vi "Wind tunnel coriolis accel calc.vi"(0 "Wind tunnel streamwise heading (deg)":dbl=90.7145, 5 "Wind tunnel streamwise elevation angle (deg)":dbl, 7 "Wind tunnel latitude (deg North of equator)":dbl=51.243148, 9 "Streamwise velocity component (m/s)":dbl=2.5, 11 "Earth angular velocity (rad/s)":dbl=7.292115e-05 format="%#.4g", 12 "Earth equatorial radius (km)":dbl=6378.137 format="%#.4g", 13 "Earth polar radius (km)":dbl=6356.7523 format="%#.4g", 14 "Wind tunnel streamwise fetch L (m)":dbl=20.0) -> (3 "Streamwise direction vector":dbl[](array[numeric])=[0.009724268343721, 0.999922245850074, -0.007806462663934707] format="%#_4g", 4 "Coriolis acceleration vector (m/s^2)":dbl[](array[numeric])=[0.00036457740038985066, -3.5455241526636534e-06, 0.0] format="%#.3e", 6 "Angle of coriolis acceleration from true North (deg)":dbl=141.23977334051196 format="%.2f", 8 "Angle of coriolis acceleration from true East (deg)":dbl=90.55718529475455 format="%.2f", 10 "Induced velocity from coriolis acceleration at L (mm/s)":dbl=2.916757121095013 format="%_3g", 15 "Induced displacement from coriolis acceleration at L (mm)":dbl=11.667028484380053 format="%_3g")   [LabVIEW 2013]
uses:
  <vilib>/Analysis/_algsub.llb/Real Vector Norm.vi
  <vilib>/Analysis/baseanly.llb/Unit Vector (DBL).vi
  <vilib>/Analysis/baseanly.llb/Real Dot Product.vi
  <vilib>/Analysis/NI_AALBase.lvlib
  <vilib>/Analysis/NI_AALPro.lvlib
panel:
  out "WGS84 Earth surface gravitational acceleration (m/s^2)":dbl=9.811808032478377
  out "Earth surface tangential velocity (m/s)":dbl=290.56938190964064
  out "WGS84 Geoid radius (km)":dbl=6365.175727728627
  # "Paul Nathan 19/02/2014"
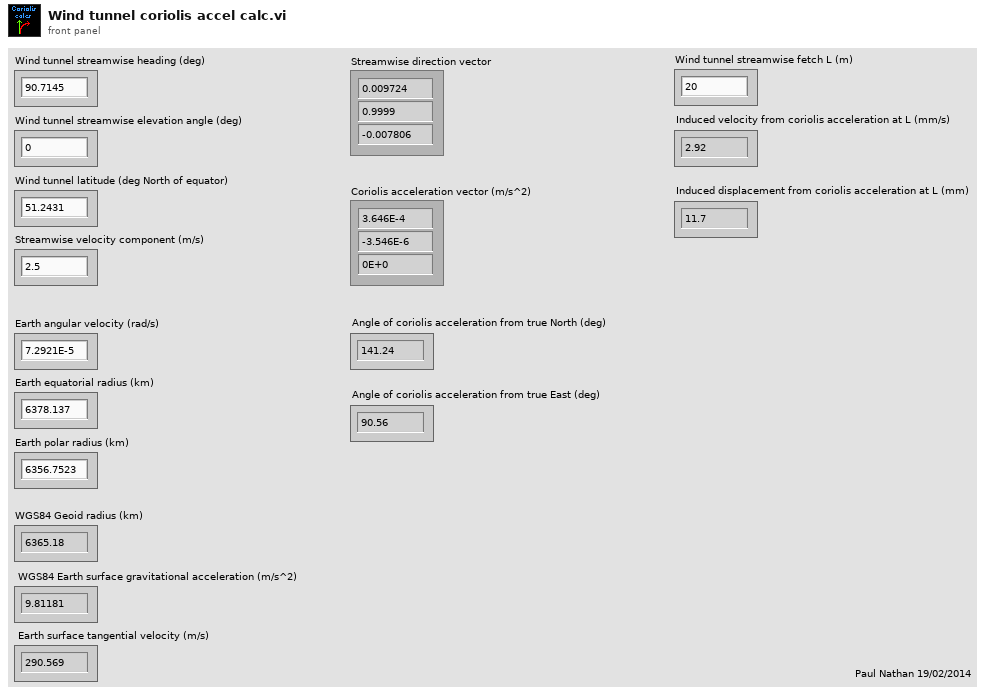
[diagram p1: front panel]
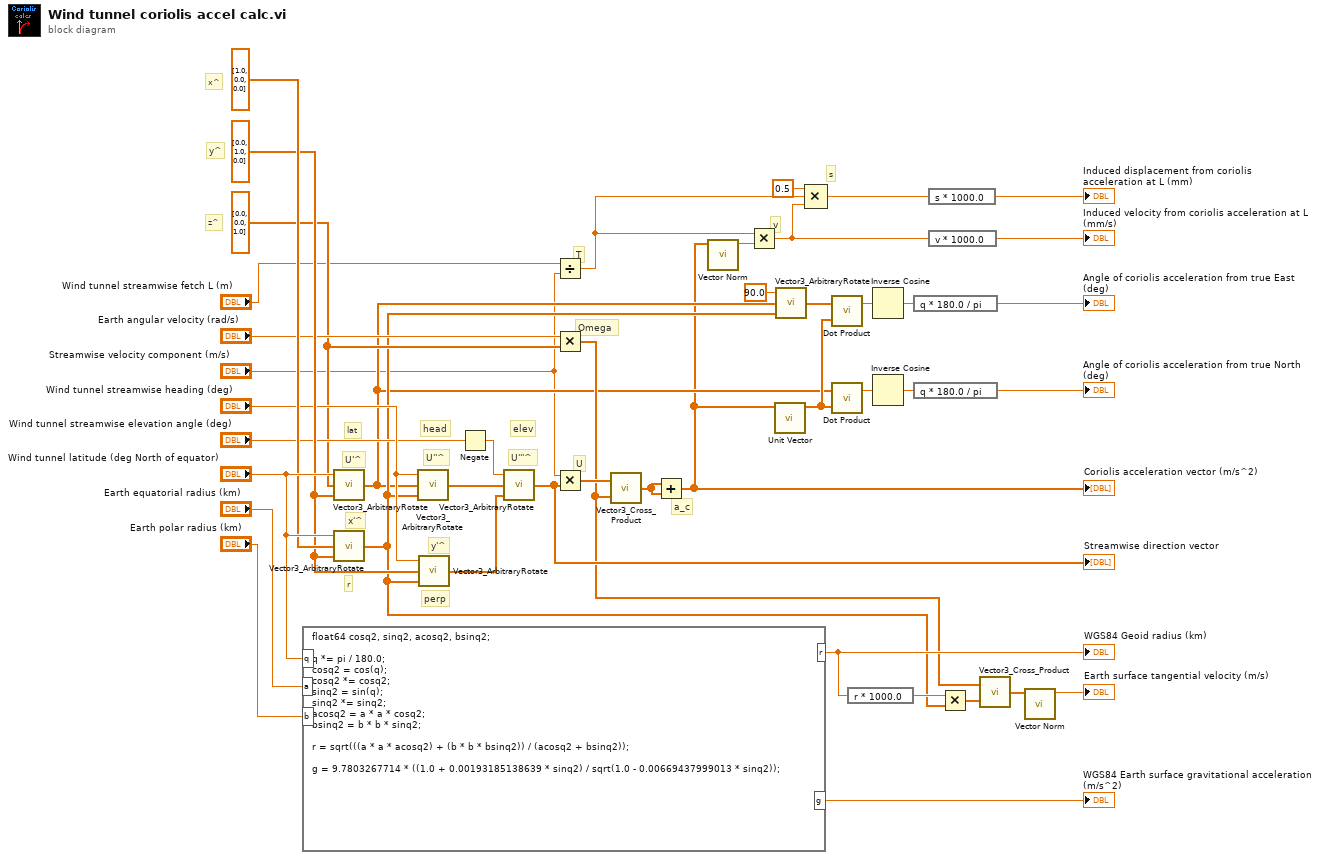
[diagram p0: block diagram]
diagram:
  w30 = dbl[] [0.0, 0.0, 1.0]
  w38 = dbl[] [0.0, 1.0, 0.0]
  # "s"
  # "v"
  # "T"
  # "U"
  # "Omega"
  # "a_c"
  # "perp"
  # "r"
  # "elev"
  # "head"
  # "lat"
  # "U'''^"
  # "y'^"
  # "U''^"
  # "x'^"
  # "U'^"
  # "x^"
  # "z^"
  # "y^"
  n1 = formula code="float64 cosq2, sinq2, acosq2, bsinq2;\n\nq *= pi / 180.0;\ncosq2 = cos(q);\ncosq2 *= cosq2;\nsinq2 = sin(q);\nsinq2 *= sinq2;\nacosq2 = a * a * cosq2;\nbsinq2 = b * b * sinq2;\n\nr = sqrt(((a * a * acosq2) + (b * b * bsinq2)) / (acosq2 + bsinq2));\n\ng = 9.7803267714 * ((1.0 + 0.00193185138639 * sinq2) / sqrt(1.0 - 0.00669437999013 * sinq2));"("q"="Wind tunnel latitude (deg North of equator)", "a"="Earth equatorial radius (km)", "b"="Earth polar radius (km)") -> ("r"=w41:dbl, "g"=→"WGS84 Earth surface gravitational acceleration (m/s^2)":dbl)
  "WGS84 Geoid radius (km)" <- w41
  n2 = call "Vector3_ArbitraryRotate.vi"("Arbitrary Axis (as UNIT Vector3)"=w38, "Input Vector3"=w30, "Rotation angle (deg)"="Wind tunnel latitude (deg North of equator)") -> ("Output Vector3"=w12:dbl[])
  n3 = call "Vector3_ArbitraryRotate.vi"("Arbitrary Axis (as UNIT Vector3)"=w38, "Input Vector3"=dbl[] [1.0, 0.0, 0.0], "Rotation angle (deg)"="Wind tunnel latitude (deg North of equator)") -> ("Output Vector3"=w13:dbl[])
  n4 = call "Vector3_ArbitraryRotate.vi"("Arbitrary Axis (as UNIT Vector3)"=w13, "Input Vector3"=w12, "Rotation angle (deg)"="Wind tunnel streamwise heading (deg)") -> ("Output Vector3"=w36:dbl[])
  n5 = call "Vector3_ArbitraryRotate.vi"("Arbitrary Axis (as UNIT Vector3)"=w13, "Input Vector3"=w38, "Rotation angle (deg)"="Wind tunnel streamwise heading (deg)") -> ("Output Vector3"=w33:dbl[])
  n6 = Negate(x="Wind tunnel streamwise elevation angle (deg)") -> (-x=w34:dbl)
  n7 = call "Vector3_ArbitraryRotate.vi"("Arbitrary Axis (as UNIT Vector3)"=w33, "Input Vector3"=w36, "Rotation angle (deg)"=w34) -> ("Output Vector3"=w28:dbl[])
  "Streamwise direction vector" <- w28
  n8 = Divide(x="Wind tunnel streamwise fetch L (m)", y="Streamwise velocity component (m/s)") -> (x/y=w6:dbl)
  n9 = Multiply(x="Earth angular velocity (rad/s)", y=w30) -> (x*y=w24:dbl[])
  n10 = Multiply(x="Streamwise velocity component (m/s)", y=w28) -> (x*y=w29:dbl[])
  n11 = call "Vector3_Cross_Product.vi"("V"=w24, "U"=w29) -> ("UxV"=w32:dbl[])
  n12 = Add(x=w32, y=w32) -> (x+y=w9:dbl[])
  "Coriolis acceleration vector (m/s^2)" <- w9
  n13 = call-poly <vilib>:"Vector Norm.vi"("Input Vector"=w9) -> ("norm"=w8:dbl)  [unwired: 9 in, 1 out]
  n14 = Multiply(x=w6, y=w8) -> (x*y=w5:dbl)
  n15 = call-poly <vilib>:"Unit Vector.vi"("Input Vector"=w9) -> ("Unit Vector"=w16:dbl[])  [unwired: 8 in, 2 out]
  n16 = call "Vector3_ArbitraryRotate.vi"("Arbitrary Axis (as UNIT Vector3)"=w13, "Input Vector3"=w12, "Rotation angle (deg)"=90.0) -> ("Output Vector3"=w15:dbl[])
  n17 = Compound Arithmetic op=MULTIPLY(0.5 ("Rotation angle (deg)"), w6, w5) -> (w4:dbl)
  n18 = call-poly <vilib>:"Dot Product.vi"("Y Vector"=w16, "X Vector"=w15) -> ("X * Y"=w17:dbl)  [unwired: 1 out]
  n19 = call-poly <vilib>:"Dot Product.vi"("Y Vector"=w16, "X Vector"=w12) -> ("X * Y"=w27:dbl)  [unwired: 1 out]
  n20 = expression code="r * 1000.0"(w41) -> (w26:dbl)
  n21 = Inverse Cosine(1:w17) -> (0:w18:dbl)
  n22 = Inverse Cosine(1:w27) -> (0:w21:dbl)
  n23 = expression code="q * 180.0 / pi"(w18) -> (→"Angle of coriolis acceleration from true East (deg)":dbl)
  n24 = expression code="q * 180.0 / pi"(w21) -> (→"Angle of coriolis acceleration from true North (deg)":dbl)
  n25 = expression code="s * 1000.0"(w4) -> (→"Induced displacement from coriolis acceleration at L (mm)":dbl)
  n26 = expression code="v * 1000.0"(w5) -> (→"Induced velocity from coriolis acceleration at L (mm/s)":dbl)
  n27 = Multiply(x=w26, y=w13) -> (x*y=w25:dbl[])
  n28 = call "Vector3_Cross_Product.vi"("V"=w25, "U"=w24) -> ("UxV"=w23:dbl[])
  n29 = call-poly <vilib>:"Vector Norm.vi"("Input Vector"=w23) -> ("norm"=→"Earth surface tangential velocity (m/s)":dbl)  [unwired: 9 in, 1 out]
